vi "Disable_stim_points_outside_stim_area.vi"(8 "error in (no error)":errorcluster, 10 "Current stim box":T1, 11 "Protocol Editor Ref IN":refnum<vi>) -> (0 "error out":errorcluster, 3 "Protocol Editor Ref OUT":refnum<vi>)   [LabVIEW 2012]
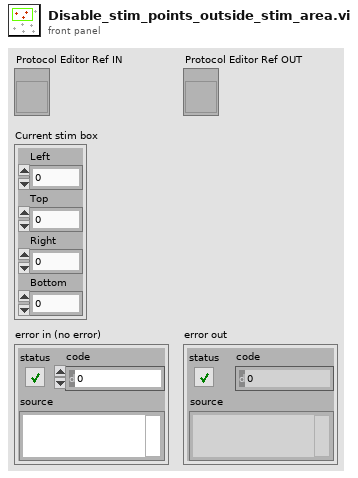
[diagram p1: front panel]
types:
  T1 = cluster{"Left":i32, "Top":i32, "Right":i32, "Bottom":i32}
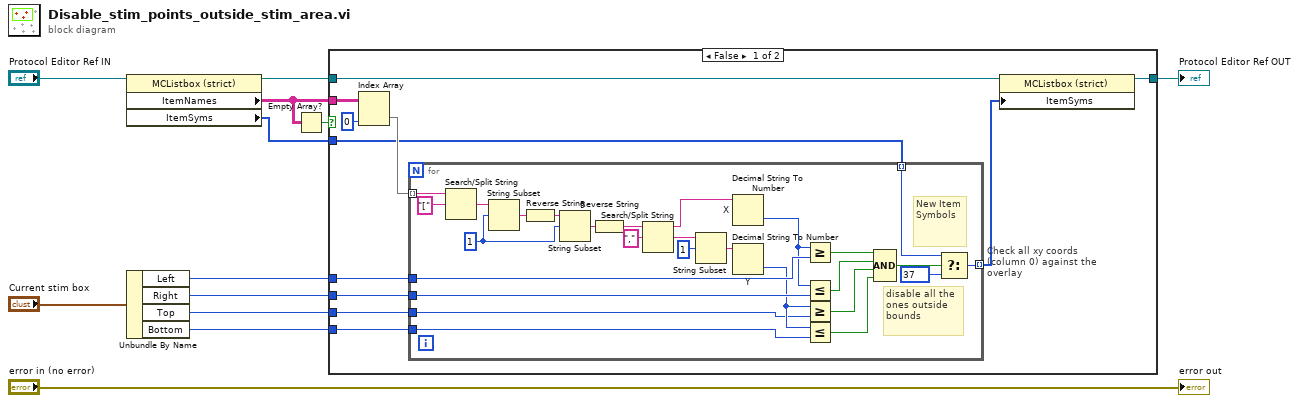
[diagram p0: block diagram]
diagram:
  n1 = property class="MCListbox (strict)"(reference="Protocol Editor Ref IN") -> (reference out=w11:refnum<vi>, "ItemNames"=w4:string[][], "ItemSyms"=w1:i32[])  [unwired: 1 in, 1 out]
  n2 = Unbundle By Name("Current stim box") -> ("Left"=w8:i32, "Right"=w7:i32, "Top"=w6:i32, "Bottom"=w5:i32)
  n3 = Empty Array?(array=w4) -> (empty?=w3:bool)
  n4 = case shown="False" w3 {
    tunnel: w11 -> [w23 w51]
    tunnel: [w22 w51] -> w10
    tunnel: w8 -> [w19 _]
    tunnel: w7 -> [w18 _]
    tunnel: w6 -> [w17 _]
    tunnel: w5 -> [w16 _]
    tunnel: w4 -> [w14 _]
    tunnel: w1 -> [w13 _]
    frame False {
      n5 = Index Array(array=w14, index (col)=0 ("disabled index (col)")) -> (element=w20:string[])  [unwired: 1 in]
      n6 = for "Check all xy coords (column 0) against the overlay" {
        tunnel: w20 -> [w38] mode=indexing
        tunnel: w19 -> [w36]
        tunnel: w18 -> [w34]
        tunnel: w17 -> [w30]
        tunnel: w16 -> [w29]
        tunnel: [w25] -> w15 mode=indexing
        tunnel: w13 -> [w24] mode=indexing
        w43 = 1 ("offset (0)")
        # "New Item Symbols"
        # "disable all the ones outside bounds"
        n7 = Search/Split String(string=w38, search string/char (-)="[") -> (match + rest of string=w40:string)  [unwired: 1 in, 2 out]
        n8 = String Subset(string=w40, offset (0)=w43) -> (substring=w41:string)  [unwired: 1 in]
        n9 = Reverse String(1:w41) -> (0:w42:string)
        n10 = String Subset(string=w42, offset (0)=w43) -> (substring=w44:string)  [unwired: 1 in]
        n11 = Reverse String(1:w44) -> (0:w45:string)
        n12 = Search/Split String(string=w45, search string/char (-)=",") -> (substring before match=w49:string, match + rest of string=w47:string)  [unwired: 1 in, 1 out]
        n13 = String Subset(string=w47, offset (0)=1) -> (substring=w50:string)  [unwired: 1 in]
        n14 = Decimal String To Number "X"(string=w49) -> (number=w35:i32)  [unwired: 2 in, 1 out]
        n15 = Decimal String To Number "Y"(string=w50) -> (number=w31:i32)  [unwired: 2 in, 1 out]
        n16 = Greater Or Equal?(x=w35, y=w36) -> (x >= y?=w33:bool)
        n17 = Less Or Equal?(x=w35, y=w34) -> (x <= y?=w32:bool)
        n18 = Greater Or Equal?(x=w31, y=w30) -> (x >= y?=w28:bool)
        n19 = Less Or Equal?(x=w31, y=w29) -> (x <= y?=w27:bool)
        n20 = Compound Arithmetic op=AND(w33, w32, w28, w27) -> (w26:bool)
        n21 = Select(t=w24, s=w26, f=37) -> (s? t:f=w25:i32)
      }
      n22 = property class="MCListbox (strict)"(reference=w23, "ItemSyms"=w15) -> (reference out=w22:refnum<vi>)  [unwired: 1 in, 1 out]
    }
    frame True {
    }
  }
  "Protocol Editor Ref OUT" <- w10
  "error out" <- "error in (no error)"
